vi "VI Tester Menu Selection.vi"(8 "error in":errorcluster, 9 "Config In":variant, 10 "Shortcut Menu Selection":T1, 11 "Active VI Info":T2) -> (0 "error out":errorcluster, 1 "Config Out":variant, 2 "Config Changed":bool)   [LabVIEW 2009]
uses:
  <vilib>/addons/_JKI Toolkits/RCF API/Right Click API.llb/Framework - Active VI Info - Cluster - __RightClickAPI.ctl
  <vilib>/addons/_JKI Toolkits/RCF API/Right Click API.llb/Framework - Selection Type - Enum - __RightClickAPI.ctl
  <vilib>/addons/_JKI Toolkits/RCF API/Right Click API.llb/Framework - Shortcut Menu Selection Events - Cluster - __RightClickAPI.ctl
  <userlib>/_OpenG.lib/array/array.llb/Filter 1D Array (String)__ogtk.vi
  <vilib>/addons/_JKI Toolkits/RCF API/Right Click API.llb/RightClickAPI.lvlib
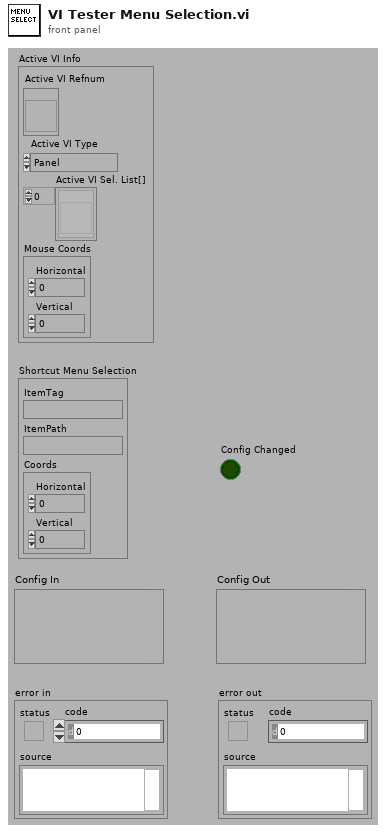
[diagram p1: front panel]
types:
  T1 = typedef "RightClickAPI.lvlib/Framework - Shortcut Menu Selection Events - Cluster - __RightClickAPI.ctl" = cluster{"ItemTag":string, "ItemPath":string, "Coords":cluster{"Horizontal":i32, "Vertical":i32}}
  T2 = typedef "RightClickAPI.lvlib/Framework - Active VI Info - Cluster - __RightClickAPI.ctl" = cluster{"Active VI Refnum":refnum<vi>, "Active VI Type":T3, "Active VI Sel. List[]":refnum<vi>[], "Mouse Coords":cluster{"Horizontal":i32, "Vertical":i32}}
  T3 = typedef "RightClickAPI.lvlib/Framework - Selection Type - Enum - __RightClickAPI.ctl" = enum16{"Panel", "Diagram"}
  T4 = cluster{"Last Test":string, "Recent Tests":string}
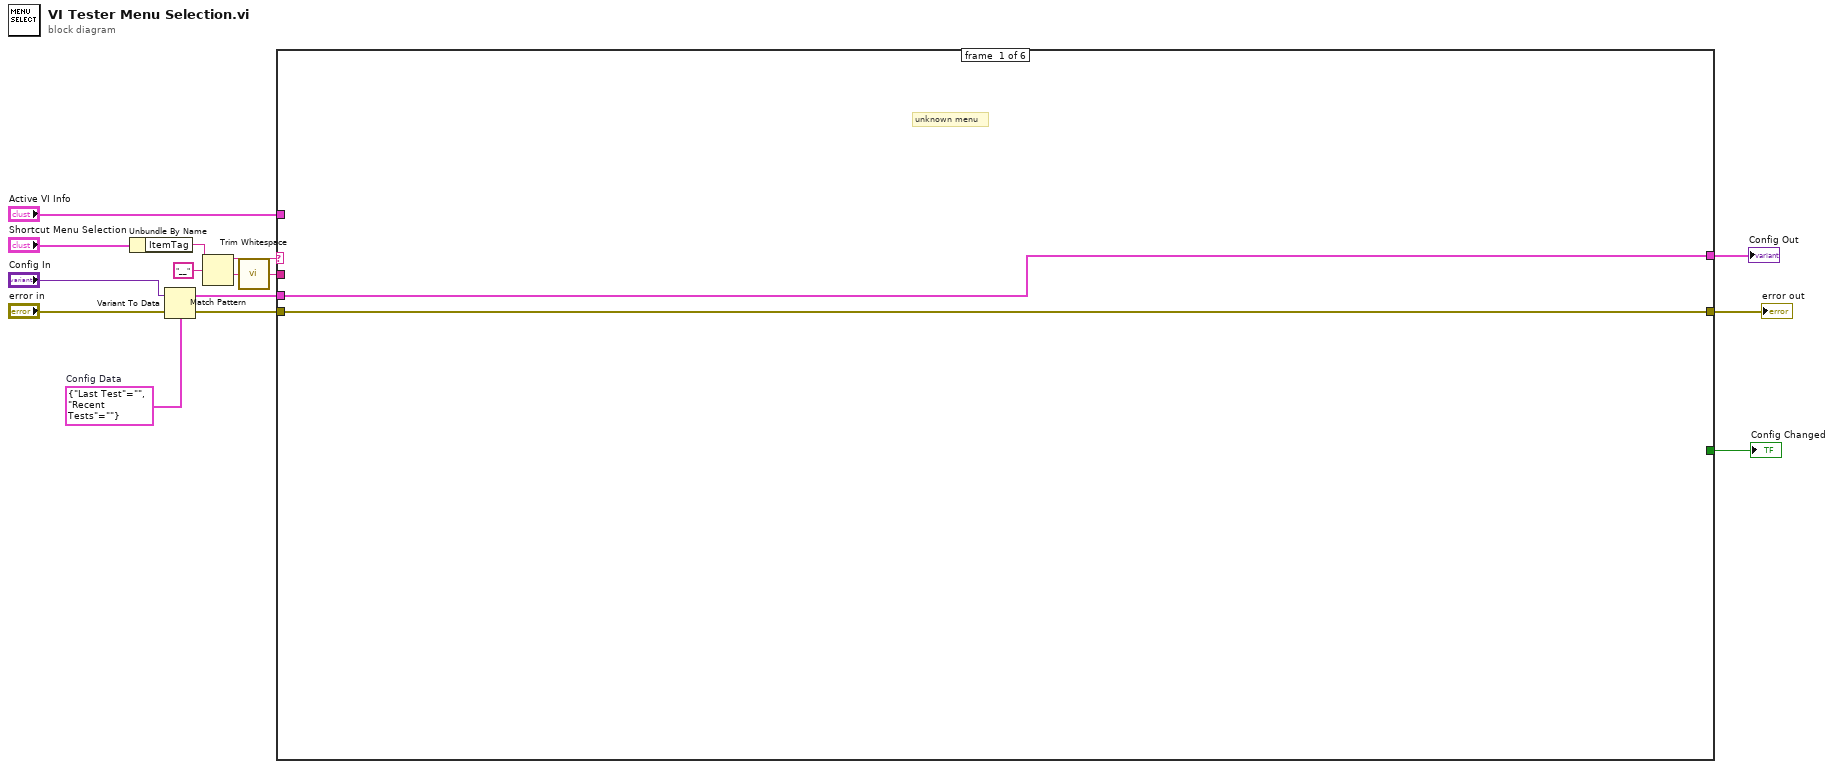
[diagram p0: block diagram]
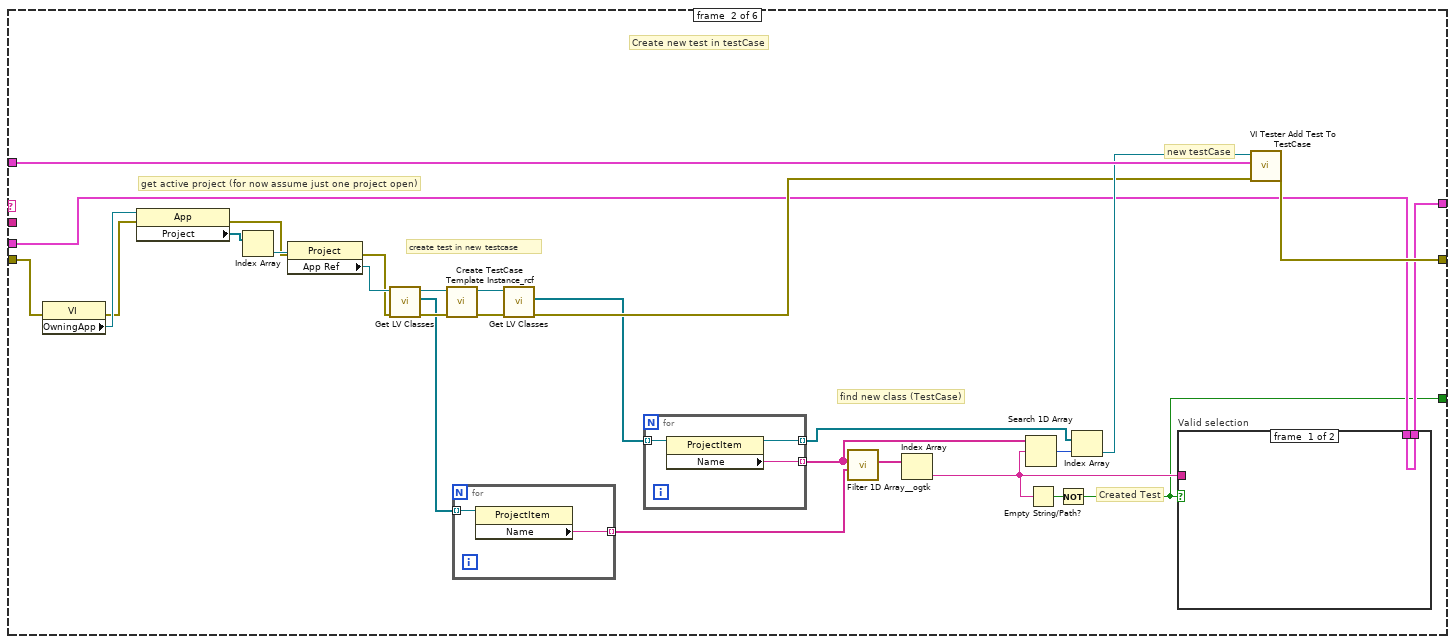
[diagram p2: hidden frame]
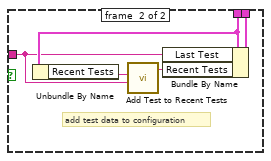
[diagram p3: hidden frame]
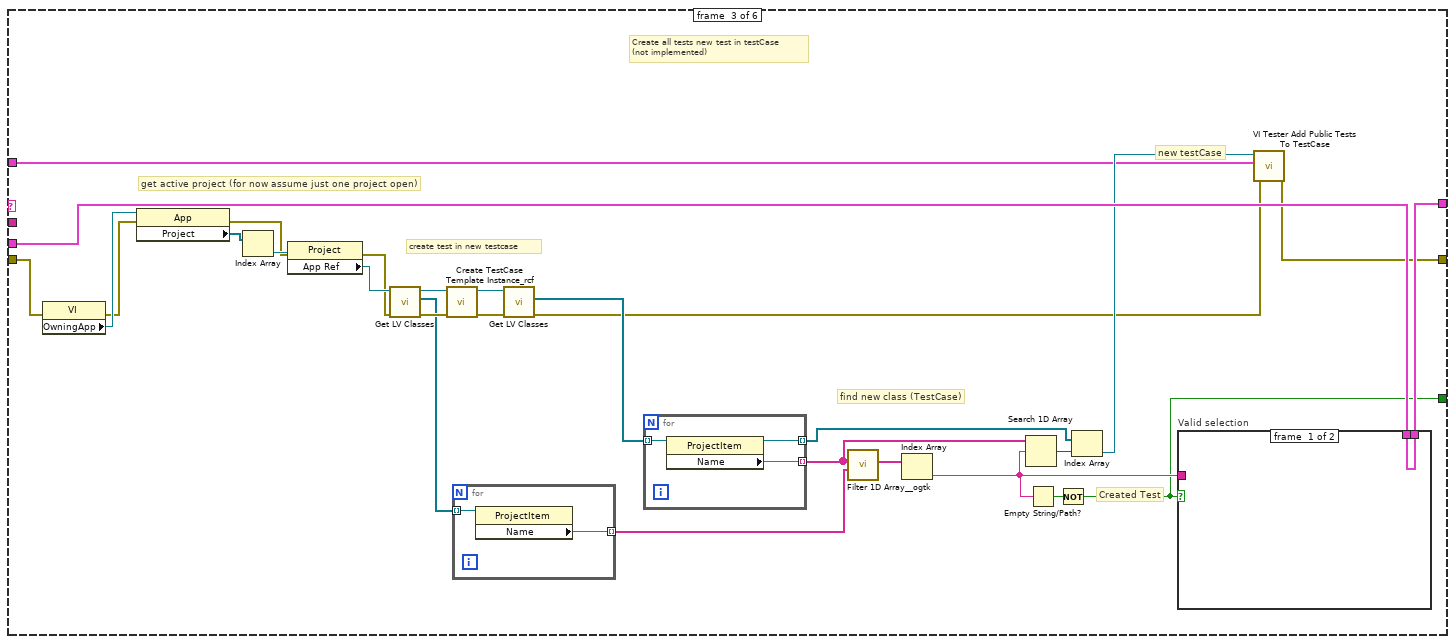
[diagram p4: hidden frame]
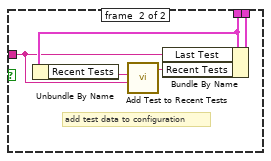
[diagram p5: hidden frame]
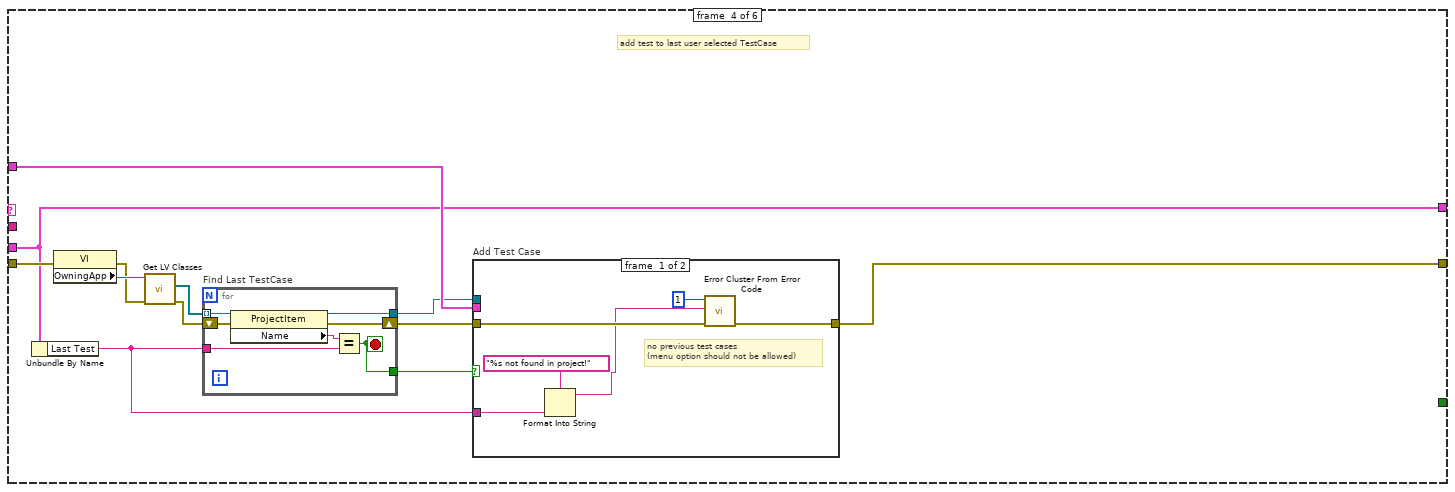
[diagram p6: hidden frame]
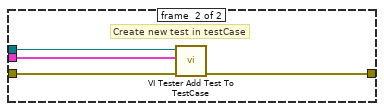
[diagram p7: hidden frame]
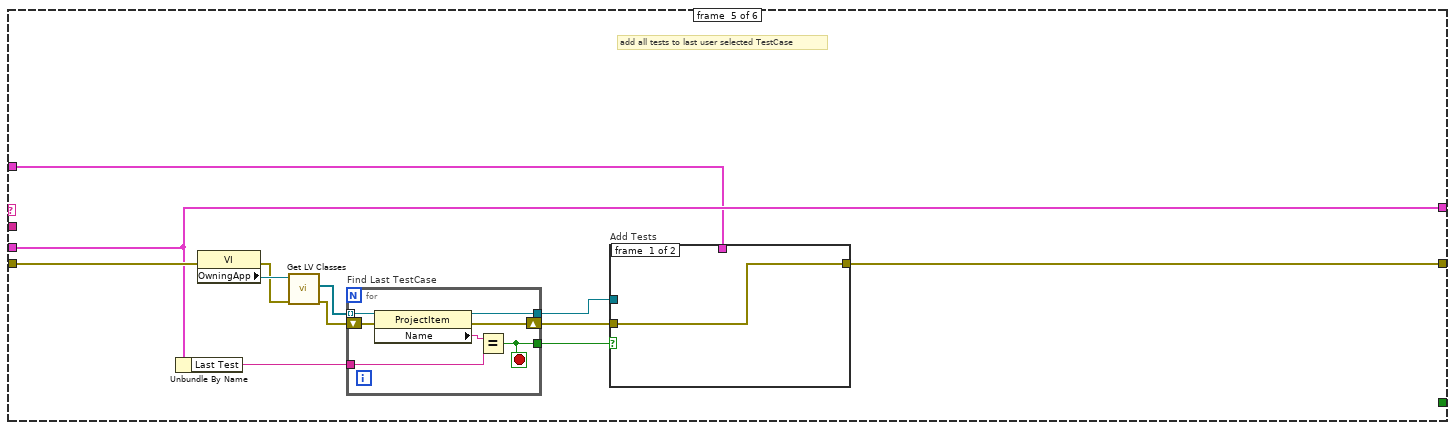
[diagram p8: hidden frame]
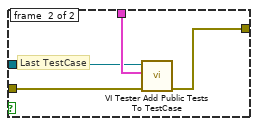
[diagram p9: hidden frame]
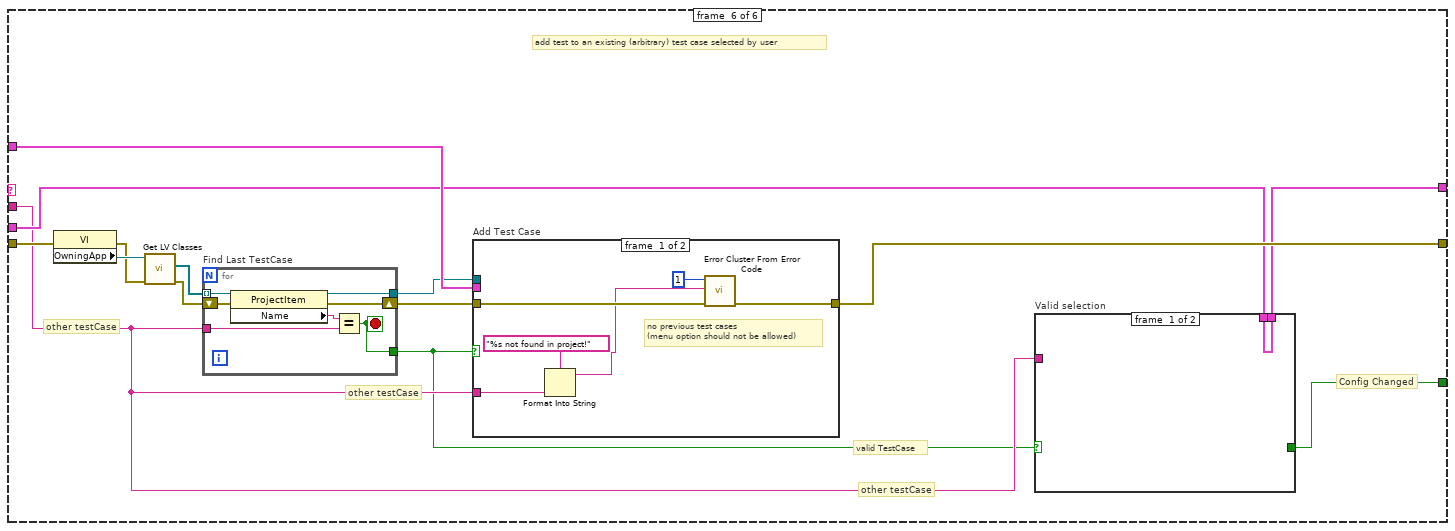
[diagram p10: hidden frame]
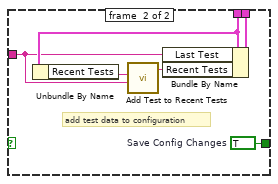
[diagram p11: hidden frame]
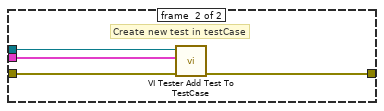
[diagram p12: hidden frame]
diagram:
  w11 = T4 {"Last Test"="", "Recent Tests"=""}  # Config Data
  n1 = Unbundle By Name("Shortcut Menu Selection") -> ("ItemTag"=w4:string)
  n2 = Variant To Data(error in="error in", Variant="Config In", type=w11) -> (error out=w9:errorcluster, data=w8:T4)
  n3 = Match Pattern(string=w4, regular expression="__") -> (before substring=w3:string, after substring=w2:string)  [unwired: 1 in, 2 out]
  n4 = call <vilib>:"Trim Whitespace.vi"("string"=w2) -> ("trimmed string"=w1:string)  [unwired: 1 in]
  n5 = case shown="\"create new test\"" w3 {
    tunnel: [w17 w44 w57 w105 w136 w160] -> w14
    tunnel: w9 -> [w17 w34 w76 w103 w134 w158]
    tunnel: "Active VI Info" -> [_ w45 w59 w107 w128 w162]
    tunnel: w8 -> [w16 w25 w68 w96 w129 w153]
    tunnel: [w16 w24 w67 w96 w129 w152] -> w7
    tunnel: [_ w21 w64 _ _ w149] -> w6
    tunnel: w1 -> [_ _ _ _ _ w151]
    frame #0 {
      # "unknown menu"
    }
    frame #1 {
      # "Created Test"
      # "Create new test in testCase"
      # "get active project (for now assume just one project open)"
      # "find new class (TestCase)"
      # "create test in new testcase"
      # "new testCase"
      n6 = property class="VI"(error in=w34) -> (error out=w19:errorcluster, "OwningApp"=w27:refnum<vi>)  [unwired: 1 in, 1 out]
      n7 = property class="App"(reference=w27, error in=w19) -> (error out=w20:errorcluster, "Project"=w29:refnum<vi>[])  [unwired: 1 out]
      n8 = Index Array(array=w29) -> (element=w28:refnum<vi>)  [unwired: 1 in]
      n9 = property class="Project"(reference=w28, error in=w20) -> (error out=w18:errorcluster, "App Ref"=w26:refnum<vi>)  [unwired: 1 out]
      n10 = call "Get LV Classes.vi"("error in (no error)"=w18, "App reference"=w26) -> ("error out"=w36:errorcluster, "LabVIEW Classes"=w32:refnum<vi>[], "dup App reference"=w30:refnum<vi>)  [unwired: 7 in]
      n11 = call "Create TestCase Template Instance_rcf.vi"("error in"=w36, "Application Ref (This Application)"=w30) -> ("error out"=w35:errorcluster, "Application Ref"=w43:refnum<vi>)  [unwired: 8 in]
      n12 = for {
        tunnel: w32 -> [w56] mode=indexing
        tunnel: [w55] -> w42 mode=indexing
        n13 = property class="ProjectItem"(reference=w56) -> ("Name"=w55:string)  [unwired: 1 in, 2 out]
      }
      n14 = call "Get LV Classes.vi"("error in (no error)"=w35, "App reference"=w43) -> ("error out"=w33:errorcluster, "LabVIEW Classes"=w31:refnum<vi>[])  [unwired: 7 in, 1 out]
      n15 = for {
        tunnel: w31 -> [w54] mode=indexing
        tunnel: [w53] -> w40 mode=indexing
        tunnel: [w52] -> w38 mode=indexing
        n16 = property class="ProjectItem"(reference=w54) -> (reference out=w52:refnum<vi>, "Name"=w53:string)  [unwired: 1 in, 1 out]
      }
      n17 = call-poly <userlib>:"Filter 1D Array__ogtk.vi"("items to filter"=w42, "array"=w40) -> ("filtered array"=w41:string[])  [unwired: 4 in, 1 out]
      n18 = Index Array(array=w41) -> (element=w23:string)  [unwired: 1 in]
      n19 = Search 1D Array(1D array=w40, element=w23) -> (index of element=w39:i32)  [unwired: 1 in]
      n20 = Empty String/Path?(string/path=w23) -> (empty?=w22:bool)
      n21 = Not(x=w22) -> (.not. x?=w21:bool)
      n22 = Index Array(array=w38, index=w39) -> (element=w37:refnum<vi>)
      n23 = case "Valid selection" shown="True" w21 {
        tunnel: w25 -> [w46 w50]
        tunnel: [w46 w51] -> w24
        tunnel: w23 -> [_ w48]
        frame #0 {
        }
        frame #1 {
          # "add test data to configuration"
          n24 = Unbundle By Name(w50) -> ("Recent Tests"=w49:string)
          n25 = call "Add Test to Recent Tests.vi"("New Test"=w48, "Recent Tests"=w49) -> ("Recent Tests"=w47:string)  [unwired: 9 in]
          n26 = Bundle By Name(cluster=w50, "Last Test"=w48, "Recent Tests"=w47) -> (w51:T4)
        }
      }
      n27 = call "VI Tester Add Test To TestCase.vi"("error in"=w33, "Active VI Info"=w45, "TestCase Refnum"=w37) -> ("error out"=w44:errorcluster)  [unwired: 8 in]
    }
    frame #2 {
      # "Created Test"
      # "Create all tests new test in testCase\n(not implemented)"
      # "get active project (for now assume just one project open)"
      # "find new class (TestCase)"
      # "create test in new testcase"
      # "new testCase"
      n28 = property class="VI"(error in=w76) -> (error out=w62:errorcluster, "OwningApp"=w70:refnum<vi>)  [unwired: 1 in, 1 out]
      n29 = property class="App"(reference=w70, error in=w62) -> (error out=w63:errorcluster, "Project"=w72:refnum<vi>[])  [unwired: 1 out]
      n30 = Index Array(array=w72) -> (element=w71:refnum<vi>)  [unwired: 1 in]
      n31 = property class="Project"(reference=w71, error in=w63) -> (error out=w61:errorcluster, "App Ref"=w69:refnum<vi>)  [unwired: 1 out]
      n32 = call "Get LV Classes.vi"("error in (no error)"=w61, "App reference"=w69) -> ("error out"=w78:errorcluster, "LabVIEW Classes"=w75:refnum<vi>[], "dup App reference"=w73:refnum<vi>)  [unwired: 7 in]
      n33 = call "Create TestCase Template Instance_rcf.vi"("error in"=w78, "Application Ref (This Application)"=w73) -> ("error out"=w77:errorcluster, "Application Ref"=w84:refnum<vi>)  [unwired: 8 in]
      n34 = for {
        tunnel: w75 -> [w95] mode=indexing
        tunnel: [w94] -> w83 mode=indexing
        n35 = property class="ProjectItem"(reference=w95) -> ("Name"=w94:string)  [unwired: 1 in, 2 out]
      }
      n36 = call "Get LV Classes.vi"("error in (no error)"=w77, "App reference"=w84) -> ("error out"=w58:errorcluster, "LabVIEW Classes"=w74:refnum<vi>[])  [unwired: 7 in, 1 out]
      n37 = for {
        tunnel: w74 -> [w93] mode=indexing
        tunnel: [w92] -> w81 mode=indexing
        tunnel: [w91] -> w79 mode=indexing
        n38 = property class="ProjectItem"(reference=w93) -> (reference out=w91:refnum<vi>, "Name"=w92:string)  [unwired: 1 in, 1 out]
      }
      n39 = call-poly <userlib>:"Filter 1D Array__ogtk.vi"("items to filter"=w83, "array"=w81) -> ("filtered array"=w82:string[])  [unwired: 4 in, 1 out]
      n40 = Index Array(array=w82) -> (element=w66:string)  [unwired: 1 in]
      n41 = Search 1D Array(1D array=w81, element=w66) -> (index of element=w80:i32)  [unwired: 1 in]
      n42 = Empty String/Path?(string/path=w66) -> (empty?=w65:bool)
      n43 = Not(x=w65) -> (.not. x?=w64:bool)
      n44 = Index Array(array=w79, index=w80) -> (element=w60:refnum<vi>)
      n45 = case "Valid selection" shown="True" w64 {
        tunnel: w68 -> [w85 w89]
        tunnel: [w85 w90] -> w67
        tunnel: w66 -> [_ w87]
        frame #0 {
        }
        frame #1 {
          # "add test data to configuration"
          n46 = Unbundle By Name(w89) -> ("Recent Tests"=w88:string)
          n47 = call "Add Test to Recent Tests.vi"("New Test"=w87, "Recent Tests"=w88) -> ("Recent Tests"=w86:string)  [unwired: 9 in]
          n48 = Bundle By Name(cluster=w89, "Last Test"=w87, "Recent Tests"=w86) -> (w90:T4)
        }
      }
      n49 = call "VI Tester Add Public Tests To TestCase.vi"("error in"=w58, "Active VI Info"=w59, "TestCase Refnum"=w60) -> ("error out"=w57:errorcluster)  [unwired: 8 in]
    }
    frame #3 {
      # "add test to last user selected TestCase"
      n50 = Unbundle By Name(w96) -> ("Last Test"=w98:string)
      n51 = property class="VI"(error in=w103) -> (error out=w102:errorcluster, "OwningApp"=w104:refnum<vi>)  [unwired: 1 in, 1 out]
      n52 = call "Get LV Classes.vi"("error in (no error)"=w102, "App reference"=w104) -> ("error out"=w101:errorcluster, "LabVIEW Classes"=w97:refnum<vi>[])  [unwired: 7 in, 1 out]
      n53 = for "Find Last TestCase" {
        tunnel: w97 -> [w124] mode=indexing
        tunnel: w98 -> [w122]
        tunnel: [w121] -> w106
        shift-right: [w119] -> w100
        shift-left: w101 -> [w120]
        tunnel: [w118] -> w99
        stop <- w118 stop-if-true
        n54 = property class="ProjectItem"(reference=w124, error in=w120) -> (reference out=w121:refnum<vi>, error out=w119:errorcluster, "Name"=w123:string)
        n55 = Equal?(x=w123, y=w122) -> (x = y?=w118:bool)
      }
      n56 = case "Add Test Case" shown="True" w99 {
        tunnel: w107 -> [_ w117]
        tunnel: w106 -> [_ w116]
        tunnel: [w112 w115] -> w105
        tunnel: w100 -> [w113 w114]
        tunnel: w98 -> [w110 _]
        frame #0 {
          # "no previous test cases\n(menu option should not be allowed)"
          n57 = Format Into String(format string="%s not found in project!", w110) -> (resulting string=w108:string)  [unwired: 2 in, 1 out]
          n58 = call <vilib>:"Error Cluster From Error Code.vi"("error in (no error)"=w113, "error message (\"\")"=w108, "error code (0)"=1) -> ("error out"=w112:errorcluster)  [unwired: 6 in]
        }
        frame #1 {
          # "Create new test in testCase"
          n59 = call "VI Tester Add Test To TestCase.vi"("error in"=w114, "Active VI Info"=w117, "TestCase Refnum"=w116) -> ("error out"=w115:errorcluster)  [unwired: 8 in]
        }
      }
    }
    frame #4 {
      # "add all tests to last user selected TestCase"
      n60 = Unbundle By Name(w129) -> ("Last Test"=w131:string)
      n61 = property class="VI"(error in=w134) -> (error out=w133:errorcluster, "OwningApp"=w135:refnum<vi>)  [unwired: 1 in, 1 out]
      n62 = call "Get LV Classes.vi"("error in (no error)"=w133, "App reference"=w135) -> ("error out"=w132:errorcluster, "LabVIEW Classes"=w130:refnum<vi>[])  [unwired: 7 in, 1 out]
      n63 = for "Find Last TestCase" {
        tunnel: w130 -> [w148] mode=indexing
        tunnel: w131 -> [w146]
        tunnel: [w145] -> w127
        shift-right: [w143] -> w126
        shift-left: w132 -> [w144]
        tunnel: [w142] -> w125
        stop <- w142 stop-if-true
        n64 = property class="ProjectItem"(reference=w148, error in=w144) -> (reference out=w145:refnum<vi>, error out=w143:errorcluster, "Name"=w147:string)
        n65 = Equal?(x=w147, y=w146) -> (x = y?=w142:bool)
      }
      n66 = case "Add Tests" shown="True" w125 {
        tunnel: [w137 w141] -> w136
        tunnel: w128 -> [_ w140]
        tunnel: w127 -> [_ w139]
        tunnel: w126 -> [w137 w138]
        frame #0 {
        }
        frame #1 {
          # "Last TestCase"
          n67 = call "VI Tester Add Public Tests To TestCase.vi"("error in"=w138, "Active VI Info"=w140, "TestCase Refnum"=w139) -> ("error out"=w141:errorcluster)  [unwired: 8 in]
        }
      }
    }
    frame #5 {
      # "add test to an existing (arbitrary) test case selected by user"
      # "Config Changed"
      # "valid TestCase"
      # "other testCase"
      # "other testCase"
      # "other testCase"
      n68 = property class="VI"(error in=w158) -> (error out=w157:errorcluster, "OwningApp"=w159:refnum<vi>)  [unwired: 1 in, 1 out]
      n69 = call "Get LV Classes.vi"("error in (no error)"=w157, "App reference"=w159) -> ("error out"=w156:errorcluster, "LabVIEW Classes"=w154:refnum<vi>[])  [unwired: 7 in, 1 out]
      n70 = for "Find Last TestCase" {
        tunnel: w154 -> [w186] mode=indexing
        tunnel: w151 -> [w184]
        tunnel: [w183] -> w161
        shift-right: [w181] -> w155
        shift-left: w156 -> [w182]
        tunnel: [w180] -> w150
        stop <- w180 stop-if-true
        n71 = property class="ProjectItem"(reference=w186, error in=w182) -> (reference out=w183:refnum<vi>, error out=w181:errorcluster, "Name"=w185:string)
        n72 = Equal?(x=w185, y=w184) -> (x = y?=w180:bool)
      }
      n73 = case "Add Test Case" shown="True" w150 {
        tunnel: w162 -> [_ w179]
        tunnel: w161 -> [_ w178]
        tunnel: [w174 w177] -> w160
        tunnel: w155 -> [w175 w176]
        tunnel: w151 -> [w172 _]
        frame #0 {
          # "no previous test cases\n(menu option should not be allowed)"
          n74 = Format Into String(format string="%s not found in project!", w172) -> (resulting string=w170:string)  [unwired: 2 in, 1 out]
          n75 = call <vilib>:"Error Cluster From Error Code.vi"("error in (no error)"=w175, "error message (\"\")"=w170, "error code (0)"=1) -> ("error out"=w174:errorcluster)  [unwired: 6 in]
        }
        frame #1 {
          # "Create new test in testCase"
          n76 = call "VI Tester Add Test To TestCase.vi"("error in"=w176, "Active VI Info"=w179, "TestCase Refnum"=w178) -> ("error out"=w177:errorcluster)  [unwired: 8 in]
        }
      }
      n77 = case "Valid selection" shown="True" w150 {
        tunnel: w153 -> [w163 w168]
        tunnel: [w163 w169] -> w152
        tunnel: w151 -> [_ w166]
        tunnel: [_ w164] -> w149
        frame #0 {
        }
        frame #1 {
          w164 = TRUE  # Save Config Changes
          # "add test data to configuration"
          n78 = Unbundle By Name(w168) -> ("Recent Tests"=w167:string)
          n79 = call "Add Test to Recent Tests.vi"("New Test"=w166, "Recent Tests"=w167) -> ("Recent Tests"=w165:string)  [unwired: 9 in]
          n80 = Bundle By Name(cluster=w168, "Last Test"=w166, "Recent Tests"=w165) -> (w169:T4)
        }
      }
    }
  }
  "error out" <- w14
  "Config Out" <- w7
  "Config Changed" <- w6
